vi "Drive Used GB.vi"(8 "error in (no error)":errorcluster, 10 "Path":path, 11 "Linux System SAL in":refnum<class "Linux System SAL.lvclass">) -> (0 "error out":errorcluster, 2 "Used GB":dbl, 3 "Linux System SAL out":refnum<class "Linux System SAL.lvclass">)   [LabVIEW 2020, in "Volatus.lvlib" / "Linux System SAL.lvclass"]
uses:
  Linux System SAL.lvclass
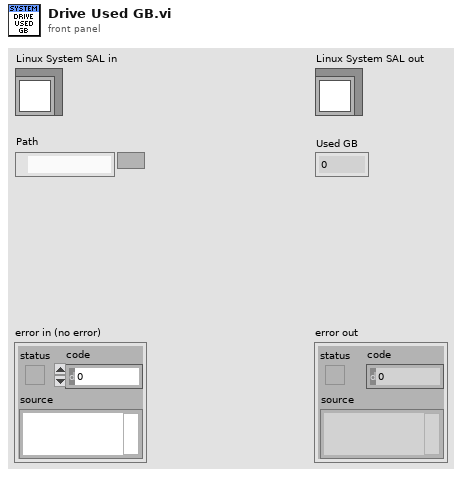
[diagram p1: front panel]
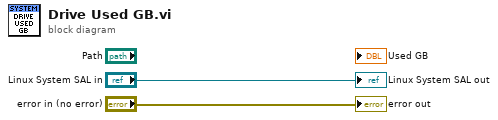
[diagram p0: block diagram]
diagram:
  "error out" <- "error in (no error)"
  "Linux System SAL out" <- "Linux System SAL in"
